vi "Select Plugin.vi"(8 "error in (no error)":errorcluster, 9 "Version String":string, 10 "Plugin Type":string="CIFTemplatePlugin", 11 "CIFPluginManager in":refnum<class "CIFPluginManager.lvclass">) -> (0 "error out":errorcluster, 1 "Match found":bool, 2 "Matching Plugin":T1, 3 "CIFPluginManager out":refnum<class "CIFPluginManager.lvclass">)   [LabVIEW 2021, in "CIFPluginManager.lvclass"]
uses:
  CIFPluginManager.lvclass
  typedef/Discovered Plugin.ctl
  CIFCore/Common/Typedef/Version.ctl
  typedef/Plugin Metadata.ctl
  CIFPluginManager.lvclass/CIFPluginManager.ctl
  CIFCore/Common/Typedef/Errors.ctl
  <vilib>/CIF Foundation/CIF Utilities/Errors/Append Error Location.vi
  CIFCore/Common/CIFCoreCommon.lvlib
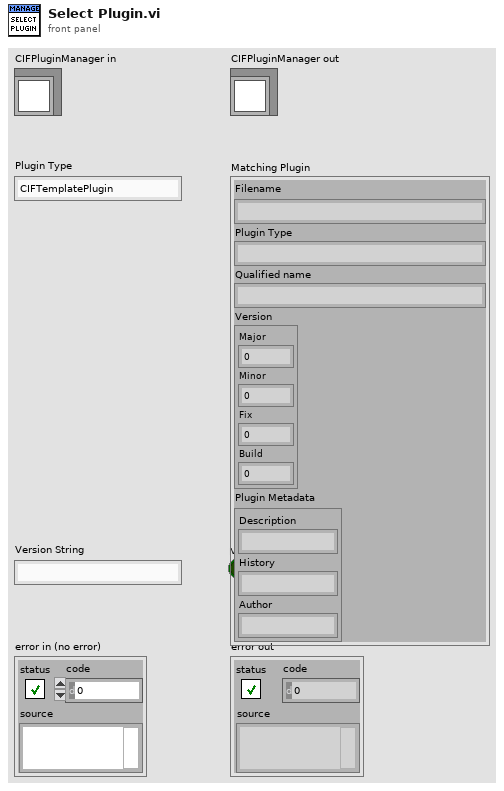
[diagram p1: front panel]
types:
  T1 = typedef "CIFPluginManager.lvclass/Discovered Plugin.ctl" = cluster{"Filename":string, "Plugin Type":string, "Qualified name":string, "Version":T2, "Plugin Metadata":T3}
  T2 = typedef "CIFCoreCommon.lvlib/Version.ctl" = cluster{"Major":i32, "Minor":i32, "Fix":i32, "Build":i32}
  T3 = typedef "CIFPluginManager.lvclass/Plugin Metadata.ctl" = cluster{"Description":string, "History":string, "Author":string}
  T4 = typedef "Discovered Plugin Map.ctl" = map{string, T1[]}
  T5 = typedef "CIFCoreCommon.lvlib/Errors.ctl" = enum16{"Invalid Clock ID", "Long Sleep", "gRPC Server Not Found", "Config Parse", "Timestamp Wrap", "Delayed Execution", "Duplicate Channel", "Missing Channel", "Incorrect Type", "Flatten Error", "Unflatten Data", "Unique Name", "Plugin Not Found", "Plugin Type Not Found", "Plugin Version Not Found", "Manager Not Found", "Numerical Issue", "Time Jump", "Clock ID Match", "Channel Length", "Plugin Connection", "gRPC Server Connection", "PPL Name Match", "Build", "Config Log Parse", "Plugin Load", "UI Subpanel Load", "Python Name", "Invalid Name", "Unable to Change Ch Buffer"}
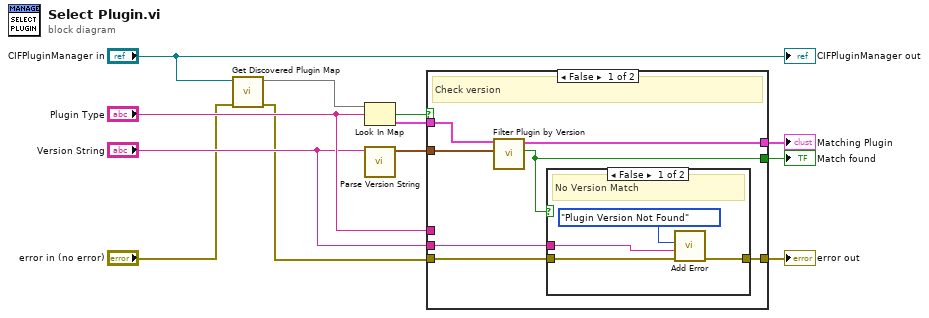
[diagram p0: block diagram]
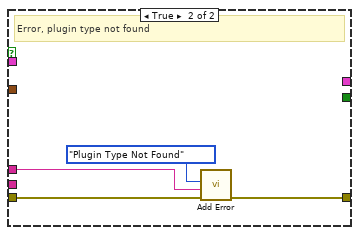
[diagram p3: hidden frame]
diagram:
  n1 = call "Get Discovered Plugin Map.vi"("error in (no error)"="error in (no error)", "CIFPluginManager in"="CIFPluginManager in") -> ("error out"=w1:errorcluster, "Discovered Plugins"=w3:T4)  [unwired: 8 in]
  n2 = Look In Map(map=w3, key="Plugin Type") -> (key not found?=w12:bool, value=w11:T1[])  [unwired: 1 in]
  n3 = call "Parse Version String.vi"("Version String"="Version String") -> ("Version"=w10:T2)  [unwired: 10 in]
  n4 = case shown="False" w12 {
    tunnel: w11 -> [w18 _]
    tunnel: w10 -> [w19 _]
    tunnel: w1 -> [w15 w28]
    tunnel: [w17 _] -> w8
    tunnel: [w16 _] -> w9
    tunnel: [w14 w27] -> w7
    tunnel: "Plugin Type" -> [_ w25]
    tunnel: "Version String" -> [w13 _]
    frame False {
      # "Check version"
      n5 = call "Filter Plugin by Version.vi"("Version Filter"=w19, "Discovered Plugins"=w18) -> ("Match found"=w16:bool, "Matching Plugin"=w17:T1)  [unwired: 8 in]
      n6 = case shown="False" w16 {
        tunnel: w15 -> [w22 w24]
        tunnel: [w23 w24] -> w14
        tunnel: w13 -> [w20 _]
        frame False {
          # "No Version Match"
          n7 = call "Add Error.vi"("error in (no error)"=w22, "String to Append"=w20, "Error"=Errors."Plugin Version Not Found") -> ("error out"=w23:errorcluster)  [unwired: 8 in]
        }
        frame True {
          # "Version Match"
        }
      }
    }
    frame True {
      # "Error, plugin type not found"
      n8 = call "Add Error.vi"("error in (no error)"=w28, "String to Append"=w25, "Error"=Errors."Plugin Type Not Found") -> ("error out"=w27:errorcluster)  [unwired: 8 in]
    }
  }
  "error out" <- w7
  "Match found" <- w9
  "Matching Plugin" <- w8
  "CIFPluginManager out" <- "CIFPluginManager in"
